vi "TCP IP Parse Read.vi"(10 "JSON in":string, 11 "Cluster in":T1) -> (2 "JSON out":string, 3 "Cluster out":T1)   [LabVIEW 2015]
panel:
  out "Energy Channel ID":string
  out "Bipolar Power Level":string
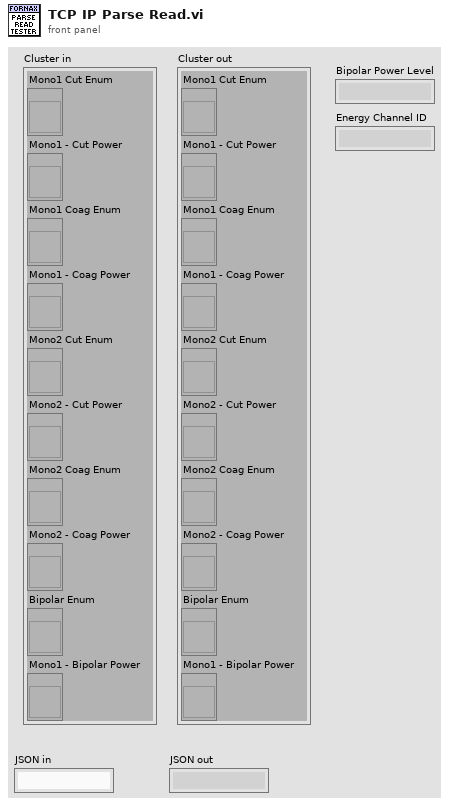
[diagram p1: front panel]
types:
  T1 = cluster{"Mono1 Cut Enum":refnum<vi>, "Mono1 - Cut Power":refnum<vi>, "Mono1 Coag Enum":refnum<vi>, "Mono1 - Coag Power":refnum<vi>, "Mono2 Cut Enum":refnum<vi>, "Mono2 - Cut Power":refnum<vi>, "Mono2 Coag Enum":refnum<vi>, "Mono2 - Coag Power":refnum<vi>, "Bipolar Enum":refnum<vi>, "Mono1 - Bipolar Power":refnum<vi>}
  T2 = typedef "Control_Fornax Bipolar Enum.ctl" = enum16{"Standard", "Macro", "Precision"}
  T3 = typedef "Control_Fornax Mono1 Cut Enum.ctl" = enum16{"Pure", "Blend"}
  T4 = typedef "Control_Fornax Mono1 Coag Enum.ctl" = enum16{"Fulgerate", "Spray"}
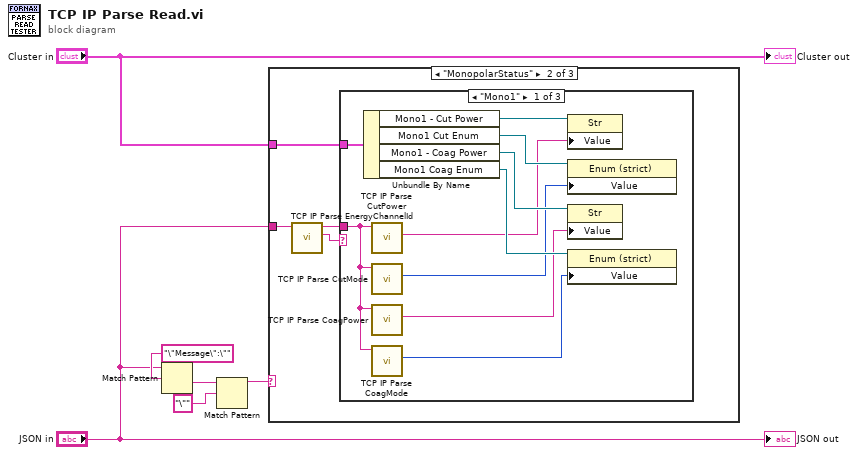
[diagram p0: block diagram]
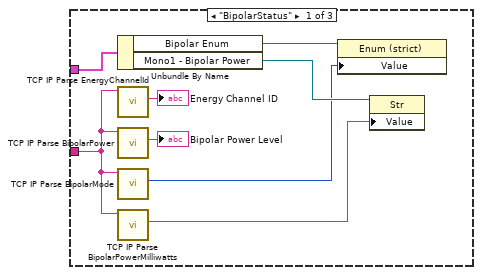
[diagram p2: hidden frame]
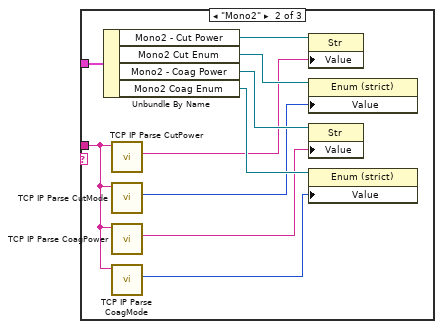
[diagram p3: hidden frame]
diagram:
  n1 = Match Pattern(string="JSON in", regular expression="\"Message\":\"") -> (after substring=w5:string)  [unwired: 1 in, 3 out]
  n2 = Match Pattern(string=w5, regular expression="\"") -> (before substring=w3:string)  [unwired: 1 in, 3 out]
  n3 = case shown="\"MonopolarStatus\"" w3 {
    tunnel: "JSON in" -> [w14 w18 _]
    tunnel: "Cluster in" -> [w12 w17 _]
    frame "BipolarStatus" {
      n4 = Unbundle By Name(w12) -> ("Bipolar Enum"=w13:refnum<vi>, "Mono1 - Bipolar Power"=w11:refnum<vi>)
      n5 = call "TCP IP Parse EnergyChannelId.vi"("JSON in"=w14) -> ("Energy Channel ID"=→"Energy Channel ID":string)  [unwired: 9 in, 1 out]
      n6 = call "TCP IP Parse BipolarPower.vi"("JSON in"=w14) -> ("Bipolar Power Level"=→"Bipolar Power Level":string)  [unwired: 9 in, 1 out]
      n7 = call "TCP IP Parse BipolarMode.vi"("JSON in"=w14) -> ("Bipolar Enum"=w7:T2)  [unwired: 9 in, 1 out]
      n8 = call "TCP IP Parse BipolarPowerMilliwatts.vi"("JSON in"=w14) -> ("Bipolar Power (xx.x)"=w10:string)  [unwired: 9 in, 1 out]
      n9 = property class="Enum (strict)"(reference=w13, "Value"=w7) -> ()  [unwired: 1 in, 2 out]
      n10 = property class="Str"(reference=w11, "Value"=w10) -> ()  [unwired: 1 in, 2 out]
    }
    frame "MonopolarStatus" {
      n11 = call "TCP IP Parse EnergyChannelId.vi"("JSON in"=w18) -> ("Energy Channel ID"=w15:string, "JSON out"=w16:string)  [unwired: 9 in]
      n12 = case shown="\"Mono1\"" w15 {
        tunnel: w17 -> [w28 w38 _]
        tunnel: w16 -> [w23 w33 _]
        frame "Mono1" {
          n13 = Unbundle By Name(w28) -> ("Mono1 - Cut Power"=w27:refnum<vi>, "Mono1 Cut Enum"=w26:refnum<vi>, "Mono1 - Coag Power"=w25:refnum<vi>, "Mono1 Coag Enum"=w24:refnum<vi>)
          n14 = call "TCP IP Parse CutPower.vi"("JSON in"=w23) -> ("Cut Power"=w22:string)  [unwired: 9 in, 1 out]
          n15 = call "TCP IP Parse CutMode.vi"("JSON in"=w23) -> ("Mono1 Cut Enum"=w21:T3)  [unwired: 9 in, 1 out]
          n16 = call "TCP IP Parse CoagPower.vi"("JSON in"=w23) -> ("Coag Power"=w20:string)  [unwired: 9 in, 1 out]
          n17 = call "TCP IP Parse CoagMode.vi"("JSON in"=w23) -> ("Mono1 Coag Enum"=w19:T4)  [unwired: 9 in, 1 out]
          n18 = property class="Str"(reference=w27, "Value"=w22) -> ()  [unwired: 1 in, 2 out]
          n19 = property class="Enum (strict)"(reference=w26, "Value"=w21) -> ()  [unwired: 1 in, 2 out]
          n20 = property class="Str"(reference=w25, "Value"=w20) -> ()  [unwired: 1 in, 2 out]
          n21 = property class="Enum (strict)"(reference=w24, "Value"=w19) -> ()  [unwired: 1 in, 2 out]
        }
        frame "Mono2" {
          n22 = Unbundle By Name(w38) -> ("Mono2 - Cut Power"=w37:refnum<vi>, "Mono2 Cut Enum"=w36:refnum<vi>, "Mono2 - Coag Power"=w35:refnum<vi>, "Mono2 Coag Enum"=w34:refnum<vi>)
          n23 = call "TCP IP Parse CutPower.vi"("JSON in"=w33) -> ("Cut Power"=w32:string)  [unwired: 9 in, 1 out]
          n24 = call "TCP IP Parse CutMode.vi"("JSON in"=w33) -> ("Mono1 Cut Enum"=w31:T3)  [unwired: 9 in, 1 out]
          n25 = call "TCP IP Parse CoagPower.vi"("JSON in"=w33) -> ("Coag Power"=w30:string)  [unwired: 9 in, 1 out]
          n26 = call "TCP IP Parse CoagMode.vi"("JSON in"=w33) -> ("Mono1 Coag Enum"=w29:T4)  [unwired: 9 in, 1 out]
          n27 = property class="Str"(reference=w37, "Value"=w32) -> ()  [unwired: 1 in, 2 out]
          n28 = property class="Enum (strict)"(reference=w36, "Value"=w31) -> ()  [unwired: 1 in, 2 out]
          n29 = property class="Str"(reference=w35, "Value"=w30) -> ()  [unwired: 1 in, 2 out]
          n30 = property class="Enum (strict)"(reference=w34, "Value"=w29) -> ()  [unwired: 1 in, 2 out]
        }
        frame Default {
        }
      }
    }
    frame "False", Default {
    }
  }
  "JSON out" <- "JSON in"
  "Cluster out" <- "Cluster in"
